vi "CircularCenter.vi"(0 "controller in":refnum<k24>, 1 "axis 1 name":string, 2 "axis 1 endpoint":dbl, 3 "axis 2 name":string, 4 "axis 2 endpoint":dbl, 5 "error in (no error)":errorcluster, 6 "speed":dbl, 7 "axis 1 center point":dbl, 8 "direction":u16(ring) items=["Clockwise", "Counter-clockwise"], 9 "axis 2 center point":dbl, 11 "return immediately":bool) -> (14 "controller out":refnum<k24>, 19 "error out":errorcluster)   [LabVIEW 2019]
uses:
  C:/Users/patrick/Documents/GitHub/Aerotech-Delay-Line/lvsrc/Aerotech-Ensemble-LabVIEW/2010-5.6/Bin/Aerotech.Ensemble.dll
  Bin/Aerotech.Ensemble.dll
  C:/Users/patrick/Documents/GitHub/Aerotech-Delay-Line/lvsrc/Aerotech-Ensemble-LabVIEW/2010-5.6/Bin/Aerotech.Ensemble.LabVIEW.dll
  Bin/Aerotech.Ensemble.LabVIEW.dll
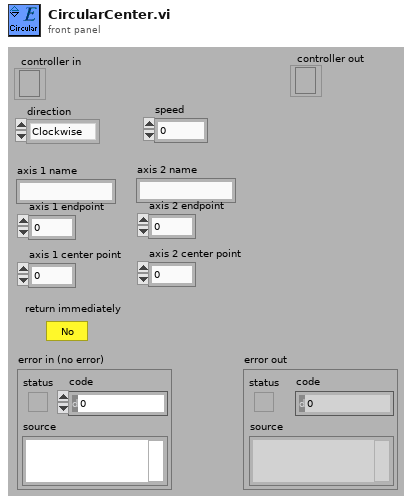
[diagram p1: front panel]
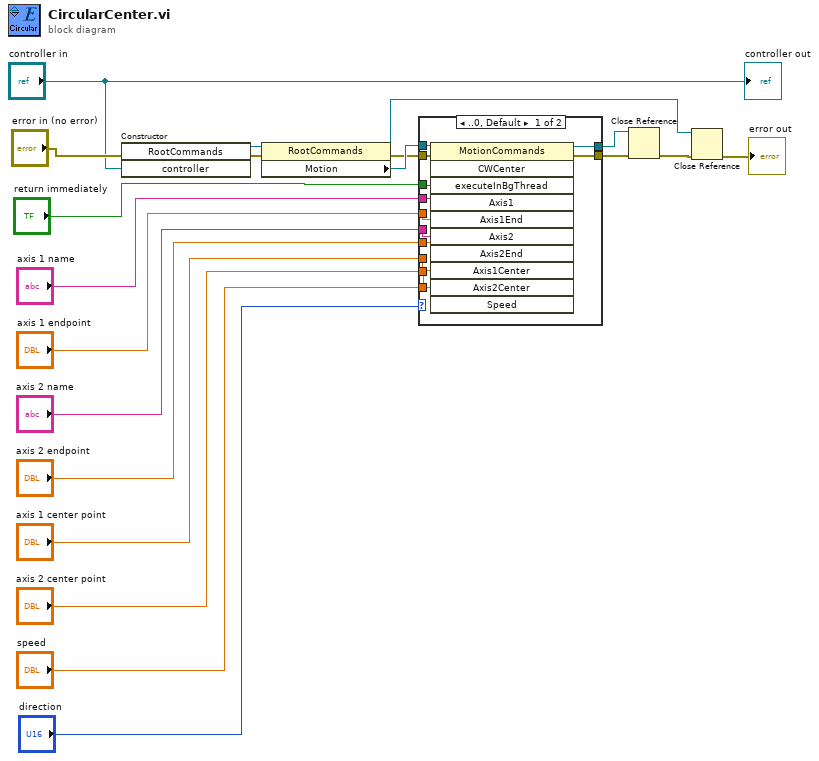
[diagram p0: block diagram]
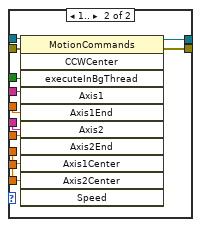
[diagram p2: hidden frame]
diagram:
  n1 = constructor class="RootCommands"(error in="error in (no error)", "controller"="controller in") -> (reference out=w6:refnum<k24>, error out=w5:errorcluster)  [unwired: 2 in, 2 out]
  n2 = property class="RootCommands"(reference=w6, error in=w5) -> (reference out=w1:refnum<k24>, error out=w7:errorcluster, "Motion"=w8:refnum<k24>)
  n3 = case shown="..0, Default" "direction" {
    tunnel: [w32 w42] -> w3
    tunnel: [w31 w41] -> w4
    tunnel: w7 -> [w30 w44]
    tunnel: w8 -> [w29 w43]
    tunnel: "speed" -> [w28 w33]
    tunnel: "axis 2 center point" -> [w27 w34]
    tunnel: "axis 1 center point" -> [w26 w35]
    tunnel: "axis 2 endpoint" -> [w25 w36]
    tunnel: "axis 2 name" -> [w24 w37]
    tunnel: "axis 1 endpoint" -> [w23 w38]
    tunnel: "axis 1 name" -> [w22 w39]
    tunnel: "return immediately" -> [w21 w40]
    frame ..0, Default {
      n4 = invoke class="MotionCommands" method="CWCenter"(reference=w29, error in=w30, "executeInBgThread"=w21, "Axis1"=w22, "Axis1End"=w23, "Axis2"=w24, "Axis2End"=w25, "Axis1Center"=w26, "Axis2Center"=w27, "Speed"=w28) -> (reference out=w32:refnum<k24>, error out=w31:errorcluster)  [unwired: 1 in, 9 out]
    }
    frame 1.. {
      n5 = invoke class="MotionCommands" method="CCWCenter"(reference=w43, error in=w44, "executeInBgThread"=w40, "Axis1"=w39, "Axis1End"=w38, "Axis2"=w37, "Axis2End"=w36, "Axis1Center"=w35, "Axis2Center"=w34, "Speed"=w33) -> (reference out=w42:refnum<k24>, error out=w41:errorcluster)  [unwired: 1 in, 9 out]
    }
  }
  n6 = Close Reference(reference=w3, error in (no error)=w4) -> (error out=w2:errorcluster)
  n7 = Close Reference(reference=w1, error in (no error)=w2) -> (error out=→"error out":errorcluster)
  "controller out" <- "controller in"
